vi "RSI6.vi"() -> ()   [LabVIEW 2018]
uses:
  <vilib>/Instr/_visa.llb/VISA Configure Serial Port (Instr).vi
panel:
  out "data out":string
  out "concatenated string":string
  out "Array":dbl[](array[numeric])
  in  "stop 2":bool
  in  "stop":bool
  out "read buffer":string
  in  "flow control (0:none)":u16(ring) items=["None", "XON/XOFF", "RTS/CTS", "XON/XOFF & RTS/CTS", "DTR/DSR", "XON/XOFF & DTR/DSR"]
  in  "stop bits (10: 1 bit)":u16(ring)=10 items=["1.0"=10, "1.5"=15, "2.0"=20]
  in  "error in (no error)":errorcluster
  in  "parity (0:none)":enum16{"None", "Odd", "Even", "Mark", "Space"}(ring)
  in  "data bits (8)":u16=8 min=5 max=8 step=1
  in  "baud rate (9600)":u32=9600
  in  "Enable Termination\nChar (T)":bool=TRUE
  in  "termination char\n(0xA = '\\n' = LF)":u8=10 format="%.0x"
  in  "timeout (10sec)":u32=10000
  in  "VISA resource name":refnum<visa-resource-name>="COM5"
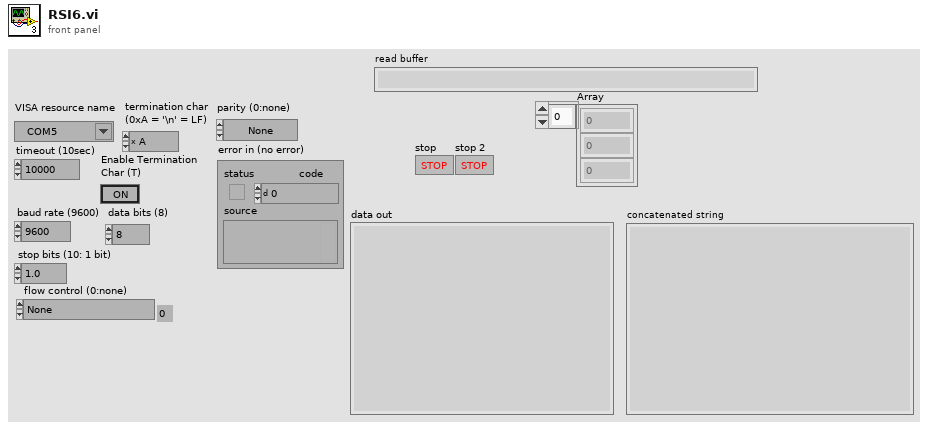
[diagram p1: front panel]
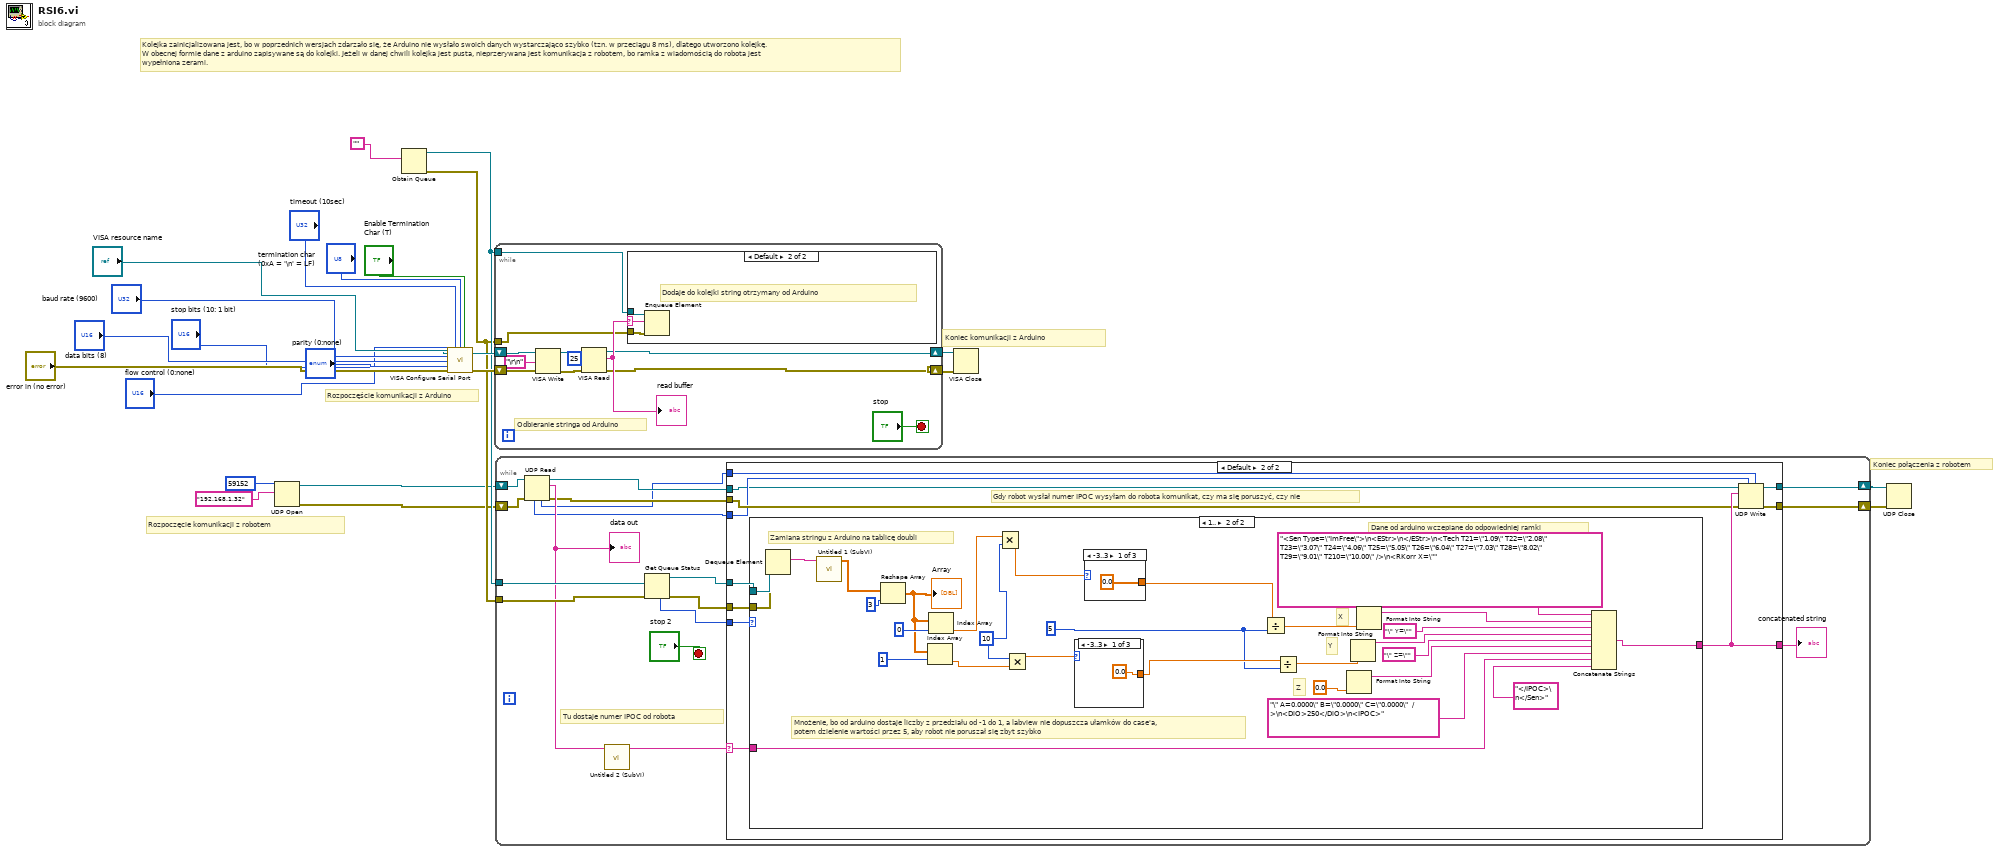
[diagram p0: block diagram]
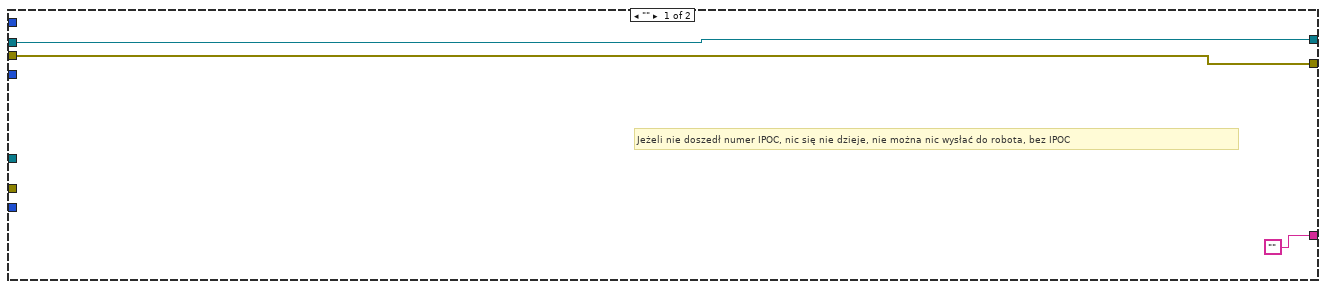
[diagram p2: hidden frame]
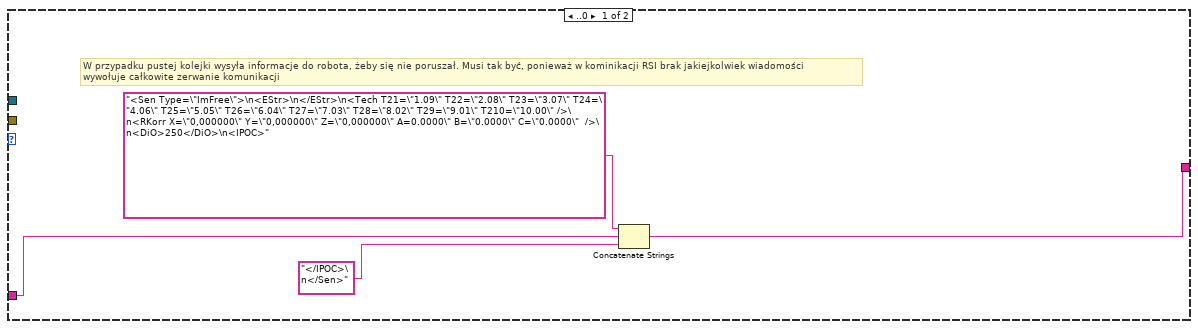
[diagram p3: hidden frame]
diagram:
  # "Kolejka zainicjalizowana jest, bo w poprzednich wersjach zdarzało się, że Arduino nie wysłało swoich danych wystarczająco szybko (tzn. w przeciągu 8 ms), dlatego utworzono kolejkę.\nW obecnej formie dane z arduino zapisywane są do kolejki. Jeżeli w danej chwili kolejka jest pusta, nieprzerywana jest komunikacja z robotem, bo ramka z wiadomością do robota jest\nwypełniona zerami."
  # "Rozpoczęście komunikacji z Arduino"
  # "Koniec komunikacji z Arduino"
  # "Rozpoczęcie komunikacji z robotem"
  # "Koniec połączenia z robotem"
  n1 = UDP Open(10:"192.168.1.32" ("service name"), 11:u16 59152 ("port")) -> (port=w9:refnum<k16>, 0:w8:errorcluster)  [unwired: 3 in, 1 out]
  n2 = Obtain Queue(element data type="") -> (queue out=w11:refnum<queue>, error out=w10:errorcluster)  [unwired: 4 in, 1 out]
  n3 = call-poly "VISA Configure Serial Port"("VISA resource name"="VISA resource name", "timeout (10sec)"="timeout (10sec)", "termination char\n(0xA = '\\n' = LF)"="termination char\n(0xA = '\\n' = LF)", "Enable Termination\nChar (T)"="Enable Termination\nChar (T)", "baud rate (9600)"="baud rate (9600)", "data bits (8)"="data bits (8)", "parity (0:none)"="parity (0:none)", "error in (no error)"="error in (no error)", "stop bits (10: 1 bit)"="stop bits (10: 1 bit)", "flow control (0:none)"="flow control (0:none)") -> ("VISA resource name out"=w13:refnum<visa-resource-name>, "error out"=w12:errorcluster)  [unwired: 4 in]
  n4 = while {
    tunnel: w11 -> [w29]
    tunnel: w10 -> [w24]
    shift-right: [w27] -> w3
    shift-left: w13 -> [w35]
    shift-right: [w26] -> w2
    shift-left: w12 -> [w34]
    stop <- "stop" stop-if-true
    # "Odbieranie stringa od Arduino"
    n5 = VISA Write(VISA resource name=w35, write buffer="\r\n", error in (no error)=w34) -> (VISA resource name out=w33:refnum<visa-resource-name>, error out=w32:errorcluster)  [unwired: 1 out]
    n6 = VISA Read(VISA resource name=w33, byte count=u32 25, error in (no error)=w32) -> (VISA resource name out=w27:refnum<visa-resource-name>, read buffer=w28:string, error out=w26:errorcluster)  [unwired: 1 out]
    "read buffer" <- w28
    n7 = case shown="Default" w28 {
      selector: w28 -> [_ w37]
      tunnel: w29 -> [_ w38]
      tunnel: w24 -> [_ w36]
      frame "" {
        # "Gdy Arduino wysyła pusty string, prawdopodobnie wystąpił błąd.\nNie ma obsługi takiego błędu, po prostu nic nie dodaje do kolejki"
      }
      frame Default {
        # "Dodaje do kolejki string otrzymany od Arduino"
        n8 = Enqueue Element(queue=w38, element=w37, error in (no error)=w36) -> ()  [unwired: 1 in, 3 out]
      }
    }
  }
  n9 = while {
    tunnel: w10 -> [w55]
    tunnel: w11 -> [w51]
    shift-right: [w42] -> w5
    shift-left: w9 -> [w49]
    shift-right: [w41] -> w4
    shift-left: w8 -> [w48]
    stop <- "stop 2" stop-if-true
    # "Tu dostaje numer IPOC od robota"
    n10 = UDP Read(connection ID=w49, 8:w48) -> (data out=w47:string, error out=w45:errorcluster, 3:w44:refnum<k16>, 4:w40:u16, 6:w39:u32)  [unwired: 2 in]
    "data out" <- w47
    n11 = call "Untitled 2 (SubVI).vi"("data in"=w47) -> ("data out"=w46:string)  [unwired: 10 in]
    n12 = Get Queue Status(queue=w51, error in (no error)=w55) -> (queue out=w54:refnum<queue>, error out=w52:errorcluster, # elements in queue=w53:i32)  [unwired: 1 in, 5 out]
    n13 = case shown="Default" w46 {
      selector: w46 -> [_ w66]
      tunnel: w54 -> [_ w69]
      tunnel: w53 -> [_ w68]
      tunnel: w52 -> [_ w67]
      tunnel: w45 -> [w57 w64]
      tunnel: w44 -> [w58 w59]
      tunnel: [w58 w63] -> w42
      tunnel: [w57 w62] -> w41
      tunnel: ["" w65] -> w43
      tunnel: w40 -> [_ w61]
      tunnel: w39 -> [_ w60]
      frame "" {
        # "Jeżeli nie doszedł numer IPOC, nic się nie dzieje, nie można nic wysłać do robota, bez IPOC"
      }
      frame Default {
        # "Gdy robot wysłał numer IPOC wysyłam do robota komunikat, czy ma się poruszyć, czy nie"
        n14 = case shown="1.." w68 {
          tunnel: w69 -> [_ w102]
          tunnel: w67 -> [_ w101]
          tunnel: w66 -> [w71 w76]
          tunnel: [w70 w75] -> w65
          frame ..0 {
            # "W przypadku pustej kolejki wysyła informacje do robota, żeby się nie poruszał. Musi tak być, ponieważ w kominikacji RSI brak jakiejkolwiek wiadomości\nwywołuje całkowite zerwanie komunikacji"
            n15 = Concatenate Strings("<Sen Type=\"ImFree\">\n<EStr>\n</EStr>\n<Tech T21=\"1.09\" T22=\"2.08\" T23=\"3.07\" T24=\"4.06\" T25=\"5.05\" T26=\"6.04\" T27=\"7.03\" T28=\"8.02\" T29=\"9.01\" T210=\"10.00\" />\n<RKorr X=\"0,000000\" Y=\"0,000000\" Z=\"0,000000\" A=0.0000\" B=\"0.0000\" C=\"0.0000\"  />\n<DiO>250</DiO>\n<IPOC>", w71, "</IPOC>\n</Sen>") -> (w70:string)
          }
          frame 1.. {
            w74 = 5
            w90 = 10
            # "Mnożenie, bo od arduino dostaje liczby z przedziału od -1 do 1, a labview nie dopuszcza ułamków do case'a,\npotem dzielenie wartości przez 5, aby robot nie poruszał się zbyt szybko"
            # "Dane od arduino wczepiane do odpowiedniej ramki"
            # "Zamiana stringu z Arduino na tablicę doubli"
            # "Z"
            # "Y"
            # "X"
            n16 = Dequeue Element(queue=w102, error in (no error)=w101) -> (element=w100:string)  [unwired: 1 in, 3 out]
            n17 = call "Untitled 1 (SubVI).vi"("String"=w100) -> ("Array"=w97:dbl[])  [unwired: 10 in]
            n18 = Reshape Array(w97, 3 ("dimension size")) -> (w95:dbl[])
            "Array" <- w95
            n19 = Index Array(array=w95, index=1) -> (element=w88:dbl)
            n20 = Index Array(array=w95, index=0) -> (element=w89:dbl)
            n21 = Multiply(x=w89, y=w90) -> (x*y=w94:dbl)
            n22 = Multiply(x=w90, y=w88) -> (x*y=w93:dbl)
            n23 = case shown="-3..3" w93 {
              selector: w93 -> [_ w107 w108]
              tunnel: [0.0 w107 w108] -> w91
              frame -3..3 {
              }
              frame ..-4 {
              }
              frame 4.. {
              }
            }
            n24 = case shown="-3..3" w94 {
              selector: w94 -> [_ w104 w105]
              tunnel: [0.0 w104 w105] -> w92
              frame -3..3 {
              }
              frame ..-4 {
              }
              frame 4.. {
              }
            }
            n25 = Divide(x=w92, y=w74) -> (x/y=w78:dbl)
            n26 = Divide(x=w91, y=w74) -> (x/y=w77:dbl)
            n27 = Format Into String(0.0 ("input 1")) -> (resulting string=w82:string)  [unwired: 3 in, 1 out]
            n28 = Format Into String(w77) -> (resulting string=w84:string)  [unwired: 3 in, 1 out]
            n29 = Format Into String(w78) -> (resulting string=w86:string)  [unwired: 3 in, 1 out]
            n30 = Concatenate Strings("<Sen Type=\"ImFree\">\n<EStr>\n</EStr>\n<Tech T21=\"1.09\" T22=\"2.08\" T23=\"3.07\" T24=\"4.06\" T25=\"5.05\" T26=\"6.04\" T27=\"7.03\" T28=\"8.02\" T29=\"9.01\" T210=\"10.00\" />\n<RKorr X=\"", w86, "\" Y=\"", w84, "\" Z=\"", w82, "\" A=0.0000\" B=\"0.0000\" C=\"0.0000\"  />\n<DiO>250</DiO>\n<IPOC>", w76, "</IPOC>\n</Sen>") -> (w75:string)
          }
        }
        n31 = UDP Write(address=w60, port or service name=w61, connection ID=w59, data in=w65, 8:w64) -> (error out=w62:errorcluster, 3:w63:refnum<k16>)  [unwired: 1 in]
      }
    }
    "concatenated string" <- w43
  }
  n32 = VISA Close(VISA resource name=w3, error in (no error)=w2) -> ()  [unwired: 1 out]
  n33 = UDP Close(connection ID=w5, 8:w4) -> ()  [unwired: 2 out]
